vi "GageTest.vi"(9 "Additional dig delay (ms) in":dbl format="%.2f", 10 "Vecchio Hitachi?":bool, 11 "Gage ID":i8=1) -> (0 "Voltage Scale (pp) OUT":i16(ring)=5, 1 "Equivalent round trip\ndelay distance (mm)":dbl format="%.2f", 3 "Output Element":T1={"Capture Config"={"Capture Mode"=0, "Sample Rate"=0, "Multiple Record"=0, "MulRec Acqs"=0}, "Input Config"={"Ch A Coupling"=0, "Ch A Input Range"=0, "Ch B Coupling"=0, "Ch B Input Range"=0}, "Trigger Config"={"Source"=0, "Slope"=0, "Coupling"=0, "Trig Input Range"=0, "Level (mV)"=0, "Trig Depth"=0}, "Transferred"={"Start Point"=0, "Number of Points"=1024, "Mulrec Group"=0}, "Vector Trigger Line"=3, "Total Delay (ms)"=0.0} {"Total Delay (ms)" format="%.2f"; "Vector Trigger Line" min=2 max=315; "Transferred"."Number of Points" min=0 max=8388608; "Transferred"."Start Point" min=-8388608 max=8388608; "Trigger Config"."Trig Depth" step=128}, 4 "Additional dig delay (ms) out":dbl format="%.2f", 5 "Total Delay (ms)":dbl format="%.2f")   [LabVIEW 2022 SP3]
uses:
  <vilib>/Analysis/NI_AALPro.lvlib
  <vilib>/Analysis/NI_AALBase.lvlib
  <vilib>/Analysis/baseanly.llb/Mean (DBL).vi
panel:
  in  "Sampling Rate":u16(ring)
  in  "Coupling 2":u16(ring) items=["DC", "AC"]
  in  "Impedance":u32=50 min=50 max=1000000 step=999950
  in  "Attenuation":u8(slide) max=63 scale=0.0..63.0
  in  "Channel":u16(ring) items=["Ch 1", "Ch 2"]
  in  "Voltage Scale (pp)":i16(ring)=5
  in  "go to scan type":bool
  in  "ExitSendCmd":bool
  in  "Coupling":u16(ring)=3 items=["DC 1 MOhm", "AC 1 MOhm", "DC 50 Ohm", "AC 50 OHM"]
  in  "Time scale per Div":i32(ring)=6 items=["100 ns", "200 ns", "500 ns", "1 micros", "2 micros", "5 micros", "10 micros", "20 micros", "50 micros", "100 micros", "500 micros", "1 ms", "5 ms", "10 ms"]
  out "Waveform\nGraph":cluster{i32, dbl, dbl[]}(graph)
  out "Error Message":string
  in  "Trigger Settings":T2={"Source"=2, "Slope"=0, "Coupling"=0, "Trig Input Range"=0, "Level (mV)"=1000, "Trig Depth"=8192, "External"=FALSE, "External Impedance"=1, "External Coupling"=0, "Source 2"=0} {"Source 2" min=0 max=64 step=1; "External Coupling" items=["DC", "AC"]; "External Impedance" items=["50 Ohm", "HiZ"]; "Trig Input Range" items=["+/- 5 Volts", "+/- 1 Volt"]; "Slope" items=["Positive", "Negative"]; "Level (mV)" min=-5000 max=5000; "Coupling" items=["DC 1 MOhm", "AC 1 MOhm"]; "Source" items=["Chan A", "Chan B", "External", "Auto"]}
  in  "RF data Sampling":T3={"Sampling Rate"=3, "Ref Delay (ms)"=0.0, "rf points per line"=2500} {"Ref Delay (ms)" format="%.2f"}
  # "Digitizer Settings"
  # "Scale Settings"
  # "Need to autoscale if viewing spectrum. Yellow curser used for additional delay.\nRF data is captured between yellow and red lines."
  # "© 2000-2004 Riverside Research Institute"
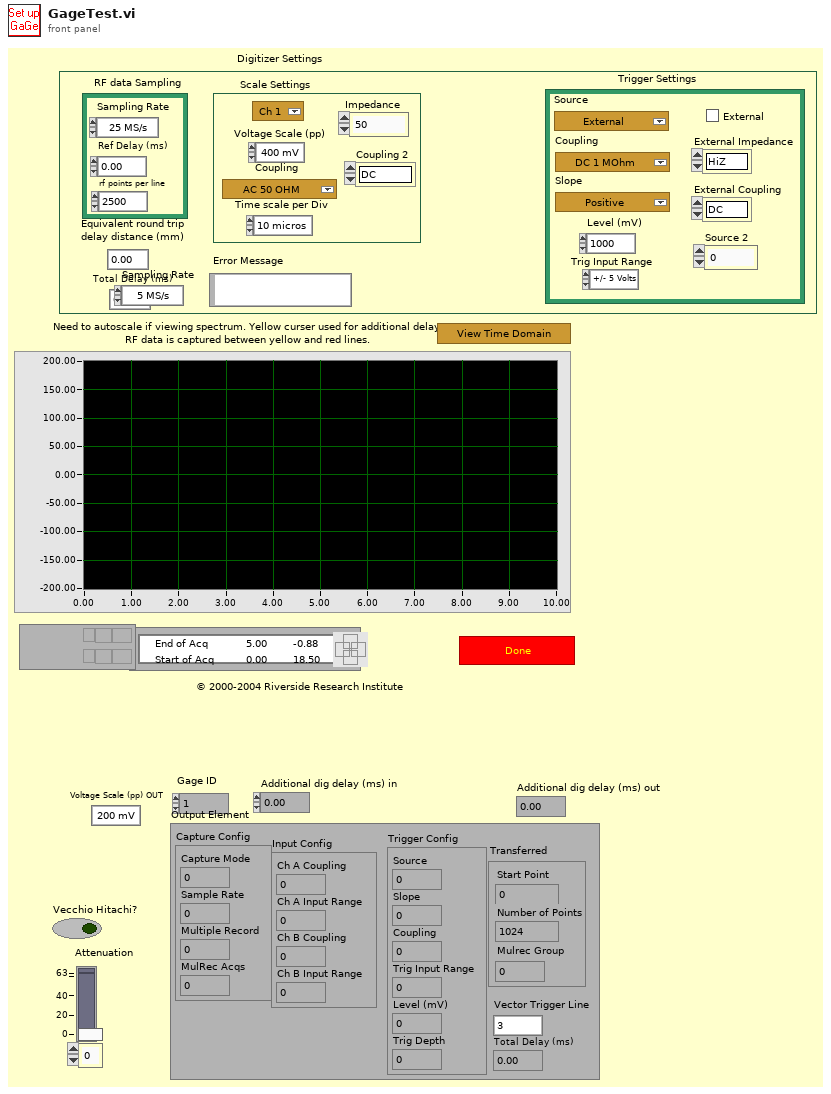
[diagram p1: front panel]
types:
  T1 = cluster{"Capture Config":cluster{"Capture Mode":i16, "Sample Rate":i32, "Multiple Record":i16, "MulRec Acqs":i16}, "Input Config":cluster{"Ch A Coupling":i16, "Ch A Input Range":i16, "Ch B Coupling":i16, "Ch B Input Range":i16}, "Trigger Config":cluster{"Source":u16, "Slope":u16, "Coupling":u16, "Trig Input Range":i16, "Level (mV)":i16, "Trig Depth":i32}, "Transferred":cluster{"Start Point":i32, "Number of Points":i32, "Mulrec Group":i32}, "Vector Trigger Line":i16, "Total Delay (ms)":sgl}
  T2 = cluster{"Source":u16, "Slope":u16, "Coupling":u16, "Trig Input Range":i16, "Level (mV)":i16, "Trig Depth":i32, "External":bool, "External Impedance":u16, "External Coupling":u16, "Source 2":i32}
  T3 = cluster{"Sampling Rate":u16, "Ref Delay (ms)":dbl, "rf points per line":u16}
  T4 = cluster{"Start Point":i32, "Number of Points":i32, "Mulrec Group":i32}
  T5 = cluster{"Sample Rate":dbl, "Clock Mode":enum16{"Internal", "External", "Reference"}, "Mode":string, "Depth":dbl, "Segment Size":dbl, "Trigger Timeout":dbl, "Trigger Holdoff":dbl, "Trigger Delay":dbl}
  T6 = cluster{"Temp Set Up Digi Params":cluster{"Sample Rate":dbl, "Clock Mode":enum16{"Internal", "External", "Reference"}, "Mode":string, "Depth":dbl, "Segment Size":dbl, "Trigger Timeout":dbl, "Trigger Holdoff":dbl, "Trigger Delay":dbl}, "sampling rate":dbl, cluster{}, "Transferred":cluster{"Start Point":i32, "Number of Points":i32, "Mulrec Group":i32}, i32, dbl}
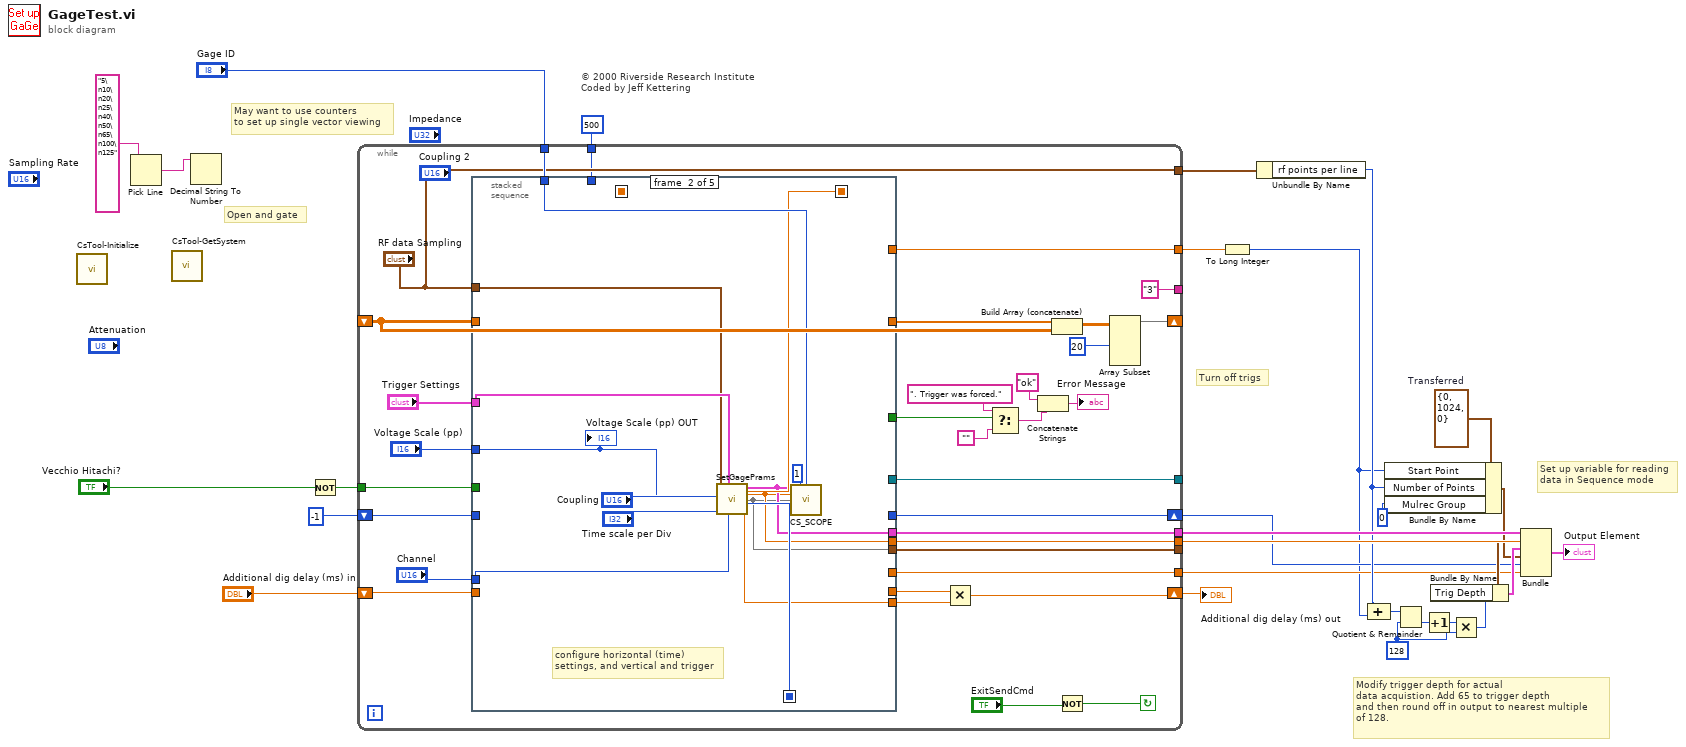
[diagram p0: block diagram]
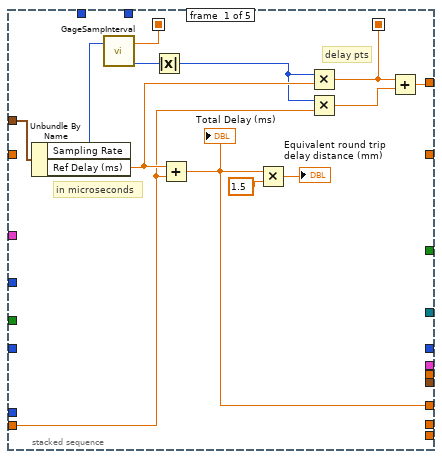
[diagram p2: hidden frame]
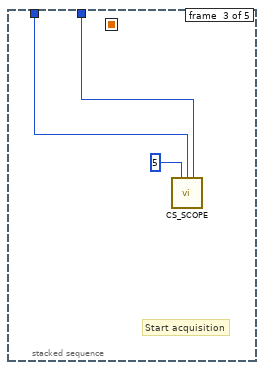
[diagram p3: hidden frame]
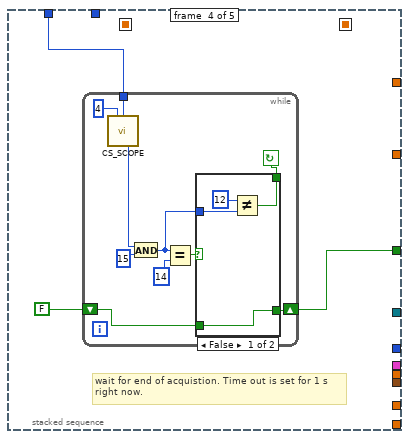
[diagram p4: hidden frame]
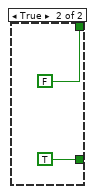
[diagram p5: hidden frame]
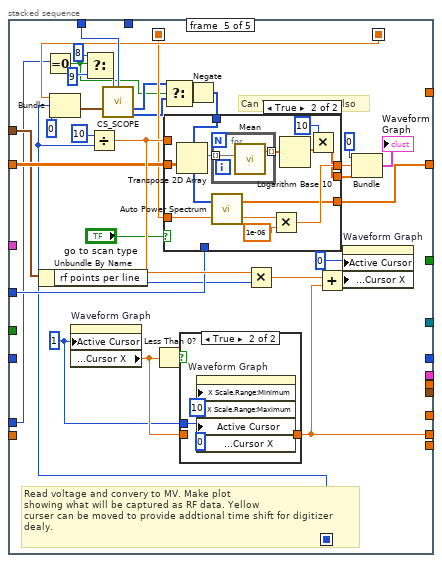
[diagram p6: hidden frame]
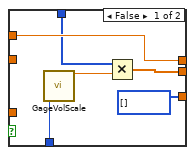
[diagram p8: hidden frame]
diagram:
  w11 = 128
  w20 = T4 {"Start Point"=0, "Number of Points"=1024, "Mulrec Group"=0}  # Transferred
  # "Open and gate"
  # "Turn off trigs"
  # "© 2000 Riverside Research Institute\nCoded by Jeff Kettering"
  # "May want to use counters\nto set up single vector viewing"
  # "Set up variable for reading\ndata in Sequence mode"
  # "Modify trigger depth for actual\ndata acquistion. Add 65 to trigger depth\nand then round off in output to nearest multiple\nof 128."
  n1 = call <userlib>:"CsTool-Initialize.vi"() -> ()  [unwired: 2 out]
  n2 = Pick Line(multi-line string="5\n10\n20\n25\n40\n50\n65\n100\n125") -> (output string=w1:string)  [unwired: 1 in, 1 out]
  n3 = call <userlib>:"CsTool-GetSystem.vi"() -> ()  [unwired: 4 in, 2 out]
  n4 = Decimal String To Number(string=w1) -> ()  [unwired: 4 out]
  n5 = Not(x="Vecchio Hitachi?") -> (.not. x?=w6:bool)
  n6 = while {
    tunnel: [w35] -> w13
    shift-left: -1 -> [w37]
    shift-right: [w36] -> w14
    tunnel: [w39] -> w22
    tunnel: [w40] -> w24
    tunnel: [w41] -> w25
    tunnel: [w42] -> w16
    tunnel: 500 -> [w43]
    shift-left: _ -> [w52]
    shift-right: [w50] -> _
    shift-left: "Additional dig delay (ms) in" -> [w53]
    shift-right: [w46] -> w30
    tunnel: ["RF data Sampling"] -> w26
    tunnel: "Gage ID" -> [w63]
    tunnel: w6 -> [w33]
    tunnel: ["3" ("counter")] -> w4
    tunnel: [w31] -> _
    stop <- w55 continue-if-true
    n7 = stacked-sequence {
      seq-local: [_ w85 _ _ _] -> [_ _ _ _ w123]
      seq-local: [w67 _ _ _ _] -> [_ w82 _ _ w131]
      seq-local: [w72 _ _ _ _] -> [_ _ _ _ w127]
      tunnel: w63 -> [_ w88 w93 w96 w132]
      tunnel: "RF data Sampling" -> [w74 w83 _ _ w124]
      tunnel: [_ _ _ w94 _] -> w58
      tunnel: "Trigger Settings" -> [_ w87 _ _ _]
      tunnel: w53 -> [w70 _ _ _ _]
      tunnel: w52 -> [_ _ _ _ w134]
      tunnel: [_ _ _ _ w113] -> w38
      tunnel: [_ _ _ _ w128] -> w48
      tunnel: [_ w84 _ _ _] -> w47
      tunnel: "Voltage Scale (pp)" -> [_ w78 _ _ w126]
      tunnel: w43 -> [_ _ w91 _ _]
      tunnel: [w68 _ _ _ _] -> w42
      tunnel: [_ w81 _ _ _] -> w41
      tunnel: [_ w80 _ _ _] -> w40
      tunnel: [_ w79 _ _ _] -> w39
      tunnel: w37 -> [_ _ _ _ _]
      tunnel: [_ _ _ _ _] -> w36
      tunnel: [w65 _ _ _ _] -> w35
      tunnel: "Channel" -> [_ w77 _ _ w118]
      tunnel: w33 -> [_ _ _ _ _]
      tunnel: [_ _ _ _ _] -> w31
      frame #0 {
        # "delay pts"
        # "in microseconds"
        n8 = Unbundle By Name(w74) -> ("Sampling Rate"=w73:u16, "Ref Delay (ms)"=w71:dbl)
        n9 = call "GageSampInterval.vi"("Sampling Rate"=w73) -> ("Sampling Rate (MHz)"=w69:i32, "time (s)"=w72:dbl)  [unwired: 1 out]
        n10 = Absolute Value(x=w69) -> (abs(x)=w64:i32)
        n11 = Add(x=w71, y=w70) -> (x+y=w65:dbl)
        "Total Delay (ms)" <- w65
        n12 = Multiply(x=w65, y=1.5) -> (x*y=→"Equivalent round trip\ndelay distance (mm)":dbl)
        n13 = Multiply(x=w64, y=w71) -> (x*y=w67:dbl)
        n14 = Multiply(x=w64, y=w70) -> (x*y=w66:dbl)
        n15 = Add(x=w67, y=w66) -> (x+y=w68:dbl)
      }
      frame #1 {
        # "configure horizontal (time)\nsettings, and vertical and trigger"
        n16 = call "SetGagePrams.vi"(5:w82, 6:w77, 7:w87, "Time scale per Div"="Time scale per Div", 9:"Coupling", "Channel"=w78, "RF data Sampling"=w83) -> ("Time per division"=w84:dbl, 1:w79, "sampling rate"=w80:dbl, "Temp Set Up Digi Params"=w81:T5, "Pts to take"=w85:i32)
        n17 = call "CS_SCOPE.VI"("Capture Config"=w81, "CompuScope Mode"=1, "Board Number"=w88, "Input Config"=w80, "Trigger Config"=w79) -> ()  [unwired: 2 in, 9 out]
        "Voltage Scale (pp) OUT" <- w78
      }
      frame #2 {
        # "Start acquisition"
        n18 = call "CS_SCOPE.VI"("CompuScope Mode"=5, "Board Number"=w93, "Trigger Timout"=w91) -> ()  [unwired: 4 in, 9 out]
      }
      frame #3 {
        # "wait for end of acquistion. Time out is set for 1 s\nright now."
        n19 = while {
          tunnel: w96 -> [w97]
          shift-left: FALSE -> [w104]
          shift-right: [w105] -> w94
          stop <- w106 continue-if-true
          n20 = call "CS_SCOPE.VI"("CompuScope Mode"=4, "Board Number"=w97) -> ("Status"=w103:i32)  [unwired: 5 in, 8 out]
          n21 = And(x=w103, y=15) -> (x .and. y?=w98:i32)
          n22 = Equal?(x=w98, y=14) -> (x = y?=w99:bool)
          n23 = case shown="False" w99 {
            tunnel: [w107 FALSE] -> w106
            tunnel: [w110 TRUE] -> w105
            tunnel: w104 -> [w110 _]
            tunnel: w98 -> [w108 _]
            frame False {
              n24 = Not Equal?(x=12, y=w108) -> (x != y?=w107:bool)
            }
            frame True {
            }
          }
        }
      }
      frame #4 {
        w135 = u32 1 ("Write Attribute")
        # "Can View Spectrum Also"
        # "Read voltage and convery to MV. Make plot\nshowing what will be captured as RF data. Yellow\ncurser can be moved to provide addtional time shift for digitizer\ndealy."
        n25 = Unbundle By Name(w124) -> ("rf points per line"=w122:u16)
        n26 = Equal To 0?(x=w118) -> (x = 0?=w114:bool)
        n27 = Bundle(w131, "Pts to take"=w123, 0) -> (w129:cluster{dbl, "Pts to take":i32, i32})  [unwired: 1 out]
        n28 = property on="Waveform Graph" class="WFGraph (strict)"("Active Cursor"=w135) -> ("Cursor.Cursor Position:Cursor X"=w139:dbl)  [unwired: 2 in, 2 out]
        n29 = Select(t=8, s=w114, f=9) -> (s? t:f=w119:i32)
        n30 = Divide(x=10, y=w123) -> (x/y=w142:dbl)
        n31 = call "CS_SCOPE.VI"("CompuScope Mode"=w119, "Board Number"=w132, "Transfer Request"=w129) -> ("DATA A"=w115:i16[], "DATA B"=w117:i16[])  [unwired: 4 in, 7 out]
        n32 = Less Than 0?(x=w139) -> (x < 0?=w136:bool)
        n33 = Select(t=w115, s=w114, f=w117) -> (s? t:f=w116:i16[])
        n34 = case shown="True" w136 {
          tunnel: w139 -> [w147 _]
          tunnel: [w147 w149] -> w128
          tunnel: w135 -> [_ w150]
          frame False {
          }
          frame True {
            w149 = 0
            n35 = property on="Waveform Graph" class="WFGraph (strict)"("X Scale.Range:Minimum"=w149, "X Scale.Range:Maximum"=10, "Active Cursor"=w150, "Cursor.Cursor Position:Cursor X"=w149) -> ()  [unwired: 2 in, 2 out]
          }
        }
        n36 = Negate(x=w116) -> (-x=w125:i16[])
        n37 = case shown="True" "go to scan type" {
          tunnel: [w152 w159] -> w133
          tunnel: w125 -> [w154 w158]
          tunnel: [w156 w165] -> w141
          tunnel: w142 -> [w156 _]
          tunnel: w127 -> [_ w168]
          tunnel: w134 -> [_ w164]
          tunnel: w126 -> [w155 _]
          tunnel: [i32[] [] w157] -> w113
          frame False {
            n38 = call "GageVolScale.vi"("Voltage Scale"=w155) -> ("Scaling Factor"=w153:dbl)  [unwired: 1 in, 1 out]
            n39 = Multiply(x=w154, y=w153) -> (x*y=w152:dbl[])
          }
          frame True {
            n40 = Transpose 2D Array(2D array=w164) -> (transposed array=w163:dbl[][])
            n41 = for {
              tunnel: w163 -> [w170] mode=indexing
              tunnel: [w169] -> w162 mode=indexing
              n42 = call-poly <vilib>:"Mean.vi"("X"=w170) -> ("mean"=w169:dbl)  [unwired: 1 out]
            }
            n43 = call <vilib>:"Auto Power Spectrum.vi"("dt"=w168, "Signal (V)"=w158) -> ("df"=w167:dbl, "Power Spectrum (V^2 rms)"=w157:dbl[])
            n44 = Multiply(x=w167, y=1e-06) -> (x*y=w165:dbl)
            n45 = Logarithm Base 10(1:w162) -> (0:w160:dbl[])
            n46 = Multiply(x=10, y=w160) -> (x*y=w159:dbl[])
          }
        }
        n47 = Multiply(x=w142, y=w122) -> (x*y=w138:dbl)
        n48 = Add(x=w138, y=w128) -> (x+y=w137:dbl)
        n49 = property on="Waveform Graph" class="WFGraph (strict)"("Active Cursor"=0, "Cursor.Cursor Position:Cursor X"=w137) -> ()  [unwired: 2 in, 2 out]
        n50 = Bundle(0, w141, w133) -> (→"Waveform\nGraph":cluster{i32, dbl, dbl[]})  [unwired: 1 out]
      }
    }
    n51 = Multiply(x=w48, y=w47) -> (x*y=w46:dbl)
    n52 = Select(t=". Trigger was forced.", s=w58, f="") -> (s? t:f=w60:string)
    n53 = Concatenate Strings("ok", w60) -> (→"Error Message":string)
    n54 = Build Array (concatenate)(w38, w52) -> (w51:dbl[][])
    n55 = Not(x="ExitSendCmd") -> (.not. x?=w55:bool)
    n56 = Array Subset(array=w51, length (row)=20) -> (w50:dbl[][])  [unwired: 3 in]
  }
  "Additional dig delay (ms) out" <- w30
  n57 = To Long Integer(number=w16) -> (32bit integer=w7:i32)
  n58 = Unbundle By Name(w26) -> ("rf points per line"=w17:u16)
  n59 = Compound Arithmetic op=ADD(w17, w7) -> (w9:i32)
  n60 = Bundle By Name(cluster=w20, "Start Point"=w7, "Number of Points"=w17, "Mulrec Group"=0) -> (w18:T4)
  n61 = Quotient & Remainder(x=w9, y=w11) -> (floor(x/y)=w12:i32)  [unwired: 1 out]
  n62 = Increment(x=w12) -> (x+1=w10:i32)
  n63 = Multiply(x=w10, y=w11) -> (x*y=w8:i32)
  n64 = Bundle By Name(cluster=w22, "Trig Depth"=w8) -> (w21:cluster{})
  n65 = Bundle("Temp Set Up Digi Params"=w25, "sampling rate"=w24, w21, "Transferred"=w18, w14, w13) -> (→"Output Element":T6)  [unwired: 1 out]
